vi "Configure Motor Synchronous Speed.vi"(0 "VISA resource name":refnum<visa-resource-name>, 5 "Number of Motor Poles (2)":i32=2 min=1 max=99, 11 "error in (no error)":errorcluster, 12 "Synchronization Source (1: I1)":i32(ring)=1 items=["U1", "I1", "U2", "I2", "U3", "I3", "U4", "I4", "U5", "I5", "U6", "I6"]) -> (4 "VISA resource name out":refnum<visa-resource-name>, 15 "error out":errorcluster)   [LabVIEW 2021, in "Yokogawa WT1800 Series.lvlib"]
doc: "Configures the motor synchronous speed features.\n\n<b>Note:</b>\nThis setting valid on models with the motor evaluation function (/MTR) option."
uses:
  <instrlib>/Yokogawa WT1800 Series/Yokogawa WT1800 Series.lvlib
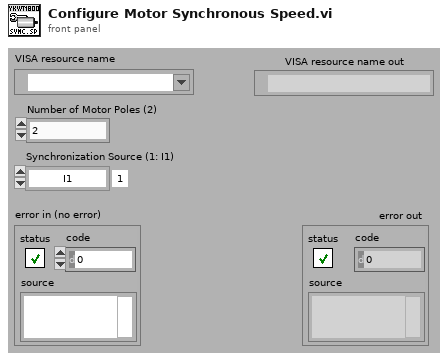
[diagram p1: front panel]
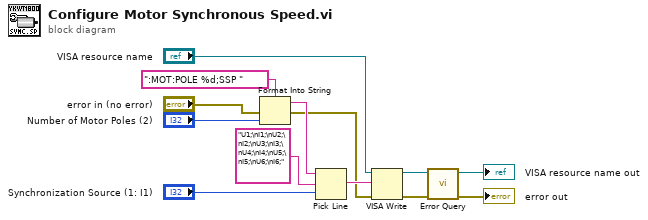
[diagram p0: block diagram]
diagram:
  n1 = Format Into String(format string=":MOT:POLE %d;SSP " ("形式文字列"), error in="error in (no error)", "Number of Motor Poles (2)") -> (resulting string=w2:string, error out=w1:errorcluster)  [unwired: 1 in]
  n2 = Pick Line ("ライン選択")(string ("")=w2, multi-line string="U1;\nI1;\nU2;\nI2;\nU3;\nI3;\nU4;\nI4;\nU5;\nI5;\nU6;\nI6;" ("複数行文字列"), line index="Synchronization Source (1: I1)") -> (output string=w4:string)
  n3 = VISA Write ("VISA書き込み")(VISA resource name="VISA resource name", write buffer=w4, error in (no error)=w1) -> (VISA resource name out=w13:refnum<visa-resource-name>, error out=w12:errorcluster)  [unwired: 1 out]
  n4 = call <instrlib>:"Error Query.vi"("error in (no error)"=w12, "VISA resource name"=w13) -> ("error out"=→"error out":errorcluster, "VISA resource name out"=→"VISA resource name out":refnum<visa-resource-name>)  [unwired: 6 in, 2 out]
